vi "DeviceOff.vi"(8 "error in (no error)":errorcluster, 11 "ChromaAcLoad in":refnum<class "ChromaAcLoad.lvclass">) -> (0 "error out":errorcluster, 3 "ChromaAcLoad out":refnum<class "ChromaAcLoad.lvclass">)   [LabVIEW 2018, in "AcPwrPlugins.lvlib" / "ChromaAcLoad.lvclass"]
doc: "This VI disable's the output of the device."
uses:
  ChromaAcLoad.lvclass
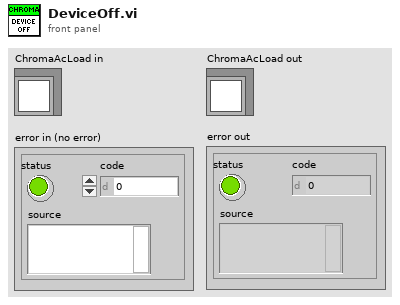
[diagram p1: front panel]
types:
  T1 = cluster{"Handle":string, "Name":string, "Phase Select":i32, "Instrument Options":string, "id query (T)":bool, "reset device (T)":bool, "Load Short Circuited":bool, "Line Synchronization":bool, "Load Current (A/Arms)":dbl, "Load Voltage (V/Vrms)":dbl, "Load Power (W)":dbl, "Load Resistance (Ohms)":dbl, "Load Current Peak Limit (A)":dbl, "Load Current Limit (A/Arms)":dbl, "Load Power Limit (W)":dbl, "Synch Frequency (Hz)":dbl, "Priority":enum16{"CF Only", "PF Only", "Both (CF)", "Both (PF)"}, "Crest Factor":dbl, "Power Factor":dbl, "Slew Rate":cluster{"Rise Slew Rate (A/ms)":i32, "Fall Slew Rate (A/ms)":i32}, "LC/RLC Mode":cluster{"Capacitance (uF)":i32, "Inductance (uH)":i32, "Series Resistance (Ohm)":dbl, "Parallel Resistance (Ohm)":dbl}, "Timing":cluster{"TimingOn":enum16{""}, "Hours":u32, "Minutes":u32, "Seconds":dbl, "CutoffVoltage":dbl}, "Connected":bool}[]
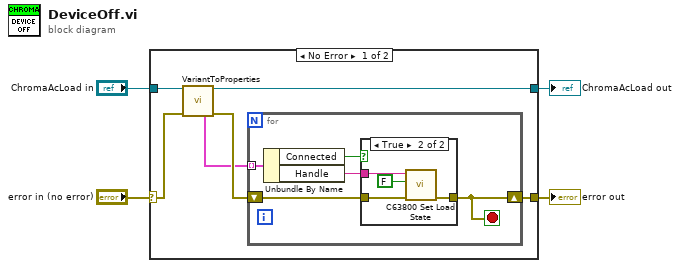
[diagram p0: block diagram]
diagram:
  n1 = case shown="No Error" "error in (no error)" {
    selector: "error in (no error)" -> [w6 w22]
    tunnel: [w10 w22] -> w2
    tunnel: [w7 w21] -> w1
    tunnel: "ChromaAcLoad in" -> [w9 w21]
    frame No Error {
      n2 = call "VariantToProperties.vi"("ChromaAcLoad"=w9, "error in (no error)"=w6) -> ("ChromaAcLoad"=w7:refnum<class "ChromaAcLoad.lvclass">, "Phases"=w5:T1, "error out"=w8:errorcluster)  [unwired: 7 in, 4 out]
      n3 = for {
        tunnel: w5 -> [w15] mode=indexing
        shift-right: [w11] -> w10
        shift-left: w8 -> [w12]
        stop <- w11 stop-if-true
        n4 = Unbundle By Name(w15) -> ("Connected"=w13:bool, "Handle"=w14:string)
        n5 = case shown="True" w13 {
          tunnel: [w16 w20] -> w11
          tunnel: w12 -> [w16 w17]
          tunnel: w14 -> [_ w18]
          frame False {
          }
          frame True, Default {
            n6 = call <instrlib>:"C63800 Set Load State.vi"("error in (no error)"=w17, "Load State"=FALSE ("Output Enabled (False)"), "Instrument Handle"=w18) -> ("error out"=w20:errorcluster)  [unwired: 7 in, 1 out]
          }
        }
      }
    }
    frame Error {
    }
  }
  "error out" <- w2
  "ChromaAcLoad out" <- w1
